vi "MTS_AutoZPos.vi"(0 "PH Dev":i32, 1 "OFlow Interv [s]":dbl, 2 "Accum Time [s]":dbl=0.1, 5 "PI System no.":i32, 11 "error in":errorcluster, 12 "Start Point":T1, 13 "Steps":i32=9, 14 "Step Width":dbl=0.1) -> (4 "New Z":dbl, 6 "Counts":u32[](array[numeric]), 15 "error out":errorcluster)   [LabVIEW 8.6]
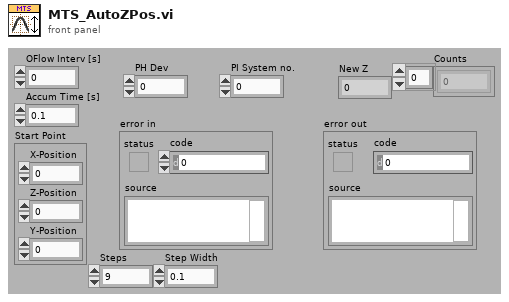
[diagram p1: front panel]
types:
  T1 = cluster{"X-Position":dbl, "Z-Position":dbl, "Y-Position":dbl}
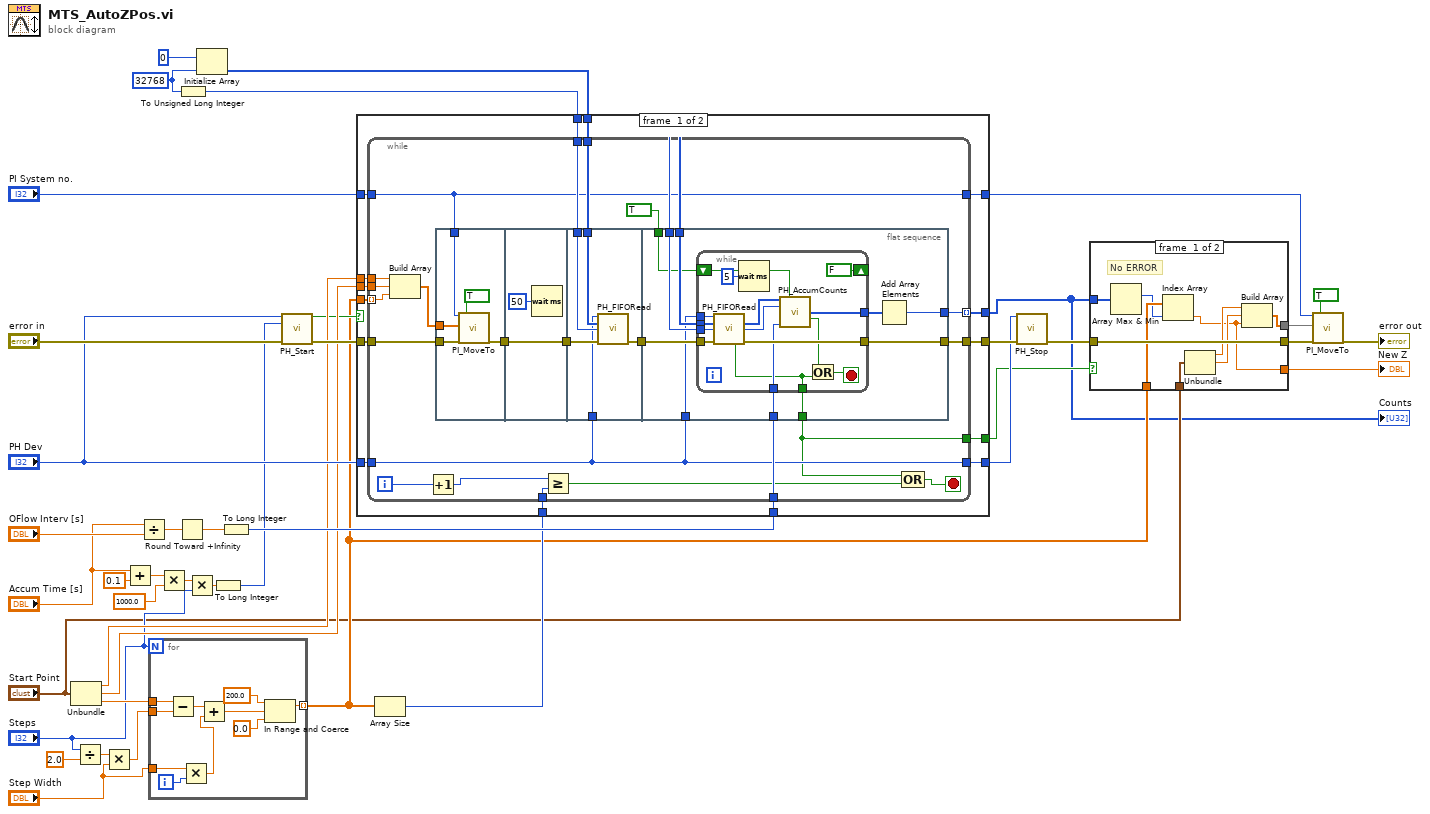
[diagram p0: block diagram]
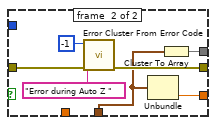
[diagram p2: hidden frame]
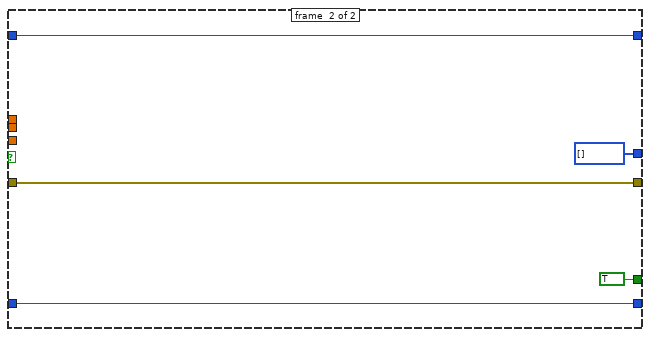
[diagram p3: hidden frame]
diagram:
  w40 = 32768 ("dimension size")
  n1 = Unbundle("Start Point") -> ("X-Position"=w21:dbl, "Z-Position"=w22:dbl, "Y-Position"=w26:dbl)
  n2 = Divide(x="Steps", y=2.0) -> (x/y=w29:dbl)
  n3 = Multiply(x=w29, y="Step Width") -> (x*y=w25:dbl)
  n4 = Add(x="Accum Time [s]", y=0.1) -> (x+y=w15:dbl)
  n5 = Divide(x="Accum Time [s]", y="OFlow Interv [s]") -> (x/y=w32:dbl)
  n6 = for {
    N: "Steps" -> [_]
    tunnel: "Step Width" -> [w51]
    tunnel: w26 -> [w50]
    tunnel: w25 -> [w47]
    tunnel: [w43] -> w5 mode=indexing
    i -> [w52]
    n7 = Subtract(x=w50, y=w47) -> (x-y=w46:dbl)
    n8 = Multiply(x=w51, y=w52) -> (x*y=w45:dbl)
    n9 = Add(x=w46, y=w45) -> (x+y=w44:dbl)
    n10 = In Range and Coerce(upper limit=200.0, x=w44, lower limit=0.0) -> (coerced(x)=w43:dbl)  [unwired: 1 out]
  }
  n11 = Multiply(x=w15, y=1000.0) -> (x*y=w13:dbl)
  n12 = Round Toward +Infinity(x=w32) -> (ceil(x): smallest int >= x=w31:dbl)
  n13 = To Unsigned Long Integer(number=w40) -> (unsigned 32bit integer=w37:u32)
  n14 = Multiply(x=w13, y="Steps") -> (x*y=w11:dbl)
  n15 = Initialize Array(u32 0, w40) -> (w38:u32[])
  n16 = To Long Integer(number=w11) -> (32bit integer=w10:i32)
  n17 = To Long Integer(number=w31) -> (32bit integer=w30:i32)
  n18 = call "PH_Start.vi"("Device Index"="PH Dev", "Acq. Time"=w10, "error in (no error)"="error in") -> ("Is Error"=w20:bool, "error out"=w41:errorcluster)  [unwired: 11 in]
  n19 = Array Size(array=w5) -> (size(s)=w23:i32)
  n20 = case shown="False" w20 {
    tunnel: w41 -> [w67 w130]
    tunnel: w38 -> [w66 _]
    tunnel: w37 -> [w65 _]
    tunnel: "PH Dev" -> [w64 w131]
    tunnel: [w63 w130] -> w35
    tunnel: "PI System no." -> [w62 w128]
    tunnel: w30 -> [w61 _]
    tunnel: [w60 w131] -> w24
    tunnel: w23 -> [w59 _]
    tunnel: w5 -> [w58 _]
    tunnel: w22 -> [w57 _]
    tunnel: w21 -> [w56 _]
    tunnel: [w55 TRUE ("FiFo Overrun")] -> w19
    tunnel: [w54 w128] -> w7
    tunnel: [w53 u32[] []] -> w1
    frame #0 {
      n21 = while {
        tunnel: w67 -> [w86]
        tunnel: w66 -> [w85]
        tunnel: w65 -> [w84]
        tunnel: w64 -> [w80]
        tunnel: [w83] -> w63
        tunnel: w62 -> [w69]
        tunnel: w61 -> [w81]
        tunnel: [w80] -> w60
        tunnel: w59 -> [w77]
        tunnel: w58 -> [w72] mode=indexing
        tunnel: w57 -> [w73]
        tunnel: w56 -> [w74]
        tunnel: [w70] -> w55
        tunnel: [w69] -> w54
        tunnel: [w68] -> w53 mode=indexing
        i -> [w79]
        stop <- w76 stop-if-true
        n22 = Build Array(w74, w73, w72) -> (w71:dbl[])
        n23 = Increment(x=w79) -> (x+1=w78:i32)
        n24 = flat-sequence {
          tunnel: w86 -> [w94]
          tunnel: [w93] -> w89
          tunnel: w69 -> [w92]
          tunnel: w71 -> [w91]
          tunnel: [w95] -> w88
          tunnel: w89 -> [w95]
          tunnel: w88 -> [w101]
          tunnel: w85 -> [w100]
          tunnel: w84 -> [w99]
          tunnel: w80 -> [w98]
          tunnel: [w97] -> w87
          tunnel: w85 -> [w110]
          tunnel: w84 -> [w109]
          tunnel: w80 -> [w108]
          tunnel: [w107] -> w83
          tunnel: w87 -> [w111]
          tunnel: TRUE ("Reset") -> [w106]
          tunnel: w81 -> [w104]
          tunnel: [w103] -> w68
          tunnel: [w102] -> w70
          frame #0 {
            n25 = call "PI_MoveTo.vi"("System no."=w92, "Target position"=w91, "error in"=w94, "Move"=TRUE) -> ("error out"=w93:errorcluster)  [unwired: 13 in, 2 out]
          }
          frame #1 {
            n26 = Wait (ms)(milliseconds to wait=u32 50) -> ()  [unwired: 1 out]
          }
          frame #2 {
            n27 = call "PH_FIFORead.vi"("Device Index"=w98, "Buffer In"=w100, "Count"=w99, "error in (no error)"=w101) -> ("error out"=w97:errorcluster)  [unwired: 7 in, 4 out]
          }
          frame #3 {
            n28 = while {
              tunnel: w111 -> [w126]
              tunnel: w110 -> [w125]
              tunnel: w109 -> [w124]
              tunnel: w108 -> [w123]
              tunnel: [w122] -> w107
              shift-right: [FALSE ("Reset")] -> _
              shift-left: w106 -> [w118]
              tunnel: [w116] -> w105
              tunnel: w104 -> [w115]
              tunnel: [w112] -> w102
              stop <- w113 stop-if-true
              n29 = call "PH_FIFORead.vi"("Device Index"=w123, "Buffer In"=w125, "Count"=w124, "error in (no error)"=w126) -> ("Buffer Out"=w120:u32[], "Data Count"=w121:i32, "FiFo Overrun"=w112:bool, "error out"=w122:errorcluster)  [unwired: 7 in, 1 out]
              n30 = Wait (ms)(milliseconds to wait=u32 5) -> ()  [unwired: 1 out]
              n31 = call "PH_AccumCounts.vi"("Data In"=w120, "Reset"=w118, "Data Count"=w121, "Acc X Overflows"=w115) -> ("Accum Counts"=w116:u32[], "Acc Time Ok"=w114:bool)  [unwired: 7 in, 3 out]
              n32 = Or(x=w114, y=w112) -> (x .or. y?=w113:bool)
            }
            n33 = Add Array Elements(numeric array=w105) -> (sum=w103:u32)
          }
        }
        n34 = Greater Or Equal?(x=w78, y=w77) -> (x >= y?=w75:bool)
        n35 = Compound Arithmetic op=OR(w70, w75) -> (w76:bool)
      }
    }
    frame #1 {
    }
  }
  "Counts" <- w1
  n36 = call "PH_Stop.vi"("Device Index"=w24, "error in (no error)"=w35) -> ("error out"=w18:errorcluster)  [unwired: 12 in, 1 out]
  n37 = case shown="False" w19 {
    tunnel: w18 -> [w140 w147]
    tunnel: [w140 w146] -> w9
    tunnel: w1 -> [w139 _]
    tunnel: w5 -> [w138 _]
    tunnel: "Start Point" -> [w136 w142]
    tunnel: [w133 w143] -> w3
    tunnel: [w132 w141] -> w2
    frame #0 {
      # "No ERROR"
      n38 = Array Max & Min(array=w139) -> (max index (indices)=w137:i32)  [unwired: 3 out]
      n39 = Index Array(array=w138, index=w137) -> (element=w132:dbl)
      n40 = Unbundle(w136) -> ("X-Position"=w135:dbl, "Z-Position"=w134:dbl)  [unwired: 1 out]
      n41 = Build Array(w135, w134, w132) -> (w133:dbl[])
    }
    frame #1 {
      n42 = call <vilib>:"Error Cluster From Error Code.vi"("error in (no error)"=w147, "error message (\"\")"="Error during Auto Z " ("error message (\"\")"), "error code (0)"=-1) -> ("error out"=w146:errorcluster)  [unwired: 6 in]
      n43 = Unbundle(w142) -> ("Y-Position"=w141:dbl)  [unwired: 2 out]
      n44 = Cluster To Array(cluster=w142) -> (array=w143:dbl[])
    }
  }
  "New Z" <- w2
  n45 = call "PI_MoveTo.vi"("System no."=w7, "Target position"=w3, "error in"=w9, "Move"=TRUE) -> ("error out"=→"error out":errorcluster)  [unwired: 13 in, 2 out]
